vi "Android_DisplayData.vi"(9 "Data Columns":string="UTC Date,UTC Time,Latitude,Longitude,Altitude,Satellites,Temperature C,Relative Humidity %,RAW H2S,RAW CH4,RAW CO\n", 11 "CSV Input":string) -> (3 "Published Data":string[][](array[string]))   [LabVIEW 2015]
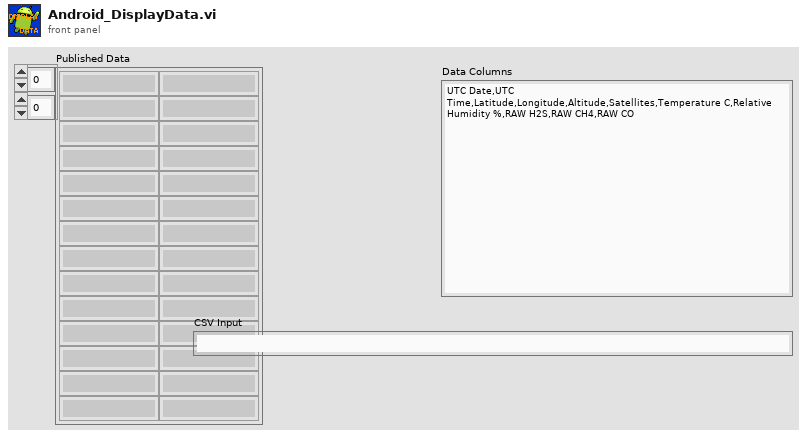
[diagram p1: front panel]
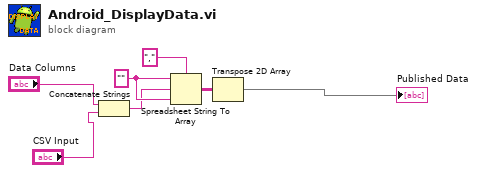
[diagram p0: block diagram]
diagram:
  w5 = "" ("format string")
  n1 = Concatenate Strings("Data Columns", "CSV Input") -> (w4:string)
  n2 = Spreadsheet String To Array(delimiter (Tab)=",", format string=w5, spreadsheet string=w4, array type (2D Dbl)=w5) -> (array=w6:string[][])
  n3 = Transpose 2D Array(2D array=w6) -> (transposed array=→"Published Data":string[][])
